vi "Launcher.vi"(8 "error in (no error)":errorcluster, 11 "Session Name":string="Session  Name") -> (0 "error out":errorcluster, 3 "VI Refnum":refnum<vi>)   [LabVIEW 2018, in "Process Bar.lvclass"]
uses:
  Process Bar.lvclass
  Utilities/UI.vi
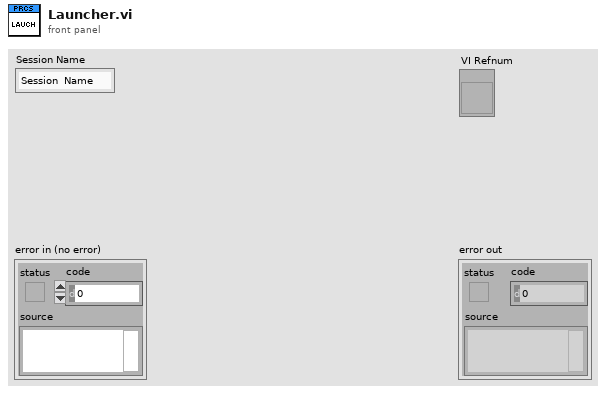
[diagram p1: front panel]
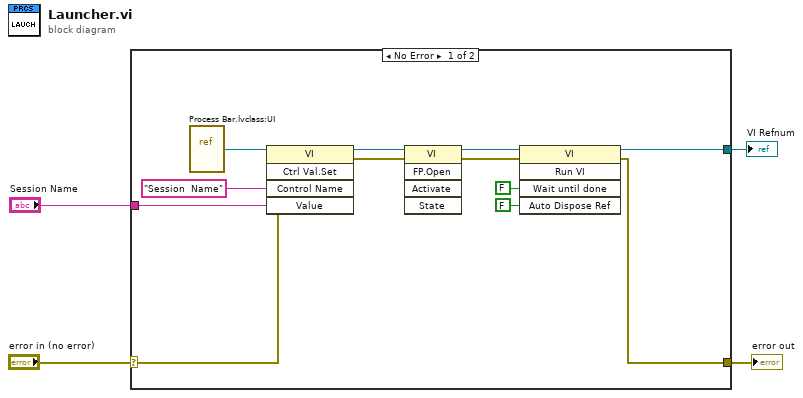
[diagram p0: block diagram]
diagram:
  n1 = case shown="No Error" "error in (no error)" {
    selector: "error in (no error)" -> [w16 w17]
    tunnel: [w6 w17] -> w3
    tunnel: "Session Name" -> [w11 _]
    tunnel: [w5 _] -> w1
    frame No Error {
      n2 = vi-ref "Process Bar.lvclass:UI.vi"() -> (w15:refnum<vi>)
      n3 = invoke class="VI" method="Ctrl Val.Set"(reference=w15, error in=w16, "Control Name"="Session  Name", "Value"=w11) -> (reference out=w10:refnum<vi>, error out=w9:errorcluster)  [unwired: 1 in, 3 out]
      n4 = invoke class="VI" method="FP.Open"(reference=w10, error in=w9) -> (reference out=w8:refnum<vi>, error out=w7:errorcluster)  [unwired: 3 in, 3 out]
      n5 = invoke class="VI" method="Run VI"(reference=w8, error in=w7, "Wait until done"=FALSE ("Wait Until Done"), "Auto Dispose Ref"=FALSE ("Auto Dispose Reference")) -> (reference out=w5:refnum<vi>, error out=w6:errorcluster)  [unwired: 1 in, 3 out]
    }
    frame Error {
    }
  }
  "error out" <- w3
  "VI Refnum" <- w1
